vi "LockFP.vi"(8 "error in (no error)":errorcluster, 11 "TektronixDPO_PhysicalDevice in":refnum<class "TektronixDPO_PhysicalDevice.lvclass">) -> (0 "error out":errorcluster, 3 "TektronixDPO_PhysicalDevice out":refnum<class "TektronixDPO_PhysicalDevice.lvclass">)   [LabVIEW 2013, in "TektronixDPO_PhysicalDevice.lvclass"]
uses:
  TektronixDPO_PhysicalDevice.lvclass
  TektronixDPO_PhysicalDevice.lvclass/TektronixDPO_PhysicalDevice.ctl
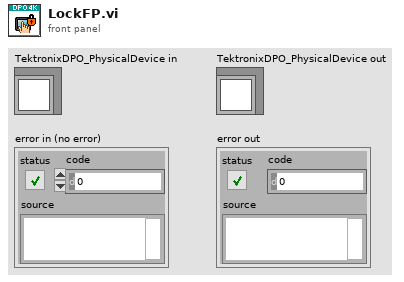
[diagram p1: front panel]
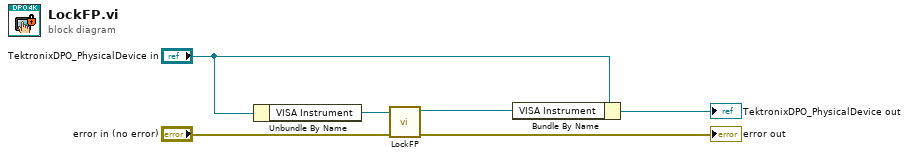
[diagram p0: block diagram]
diagram:
  n1 = Unbundle By Name("TektronixDPO_PhysicalDevice in") -> ("VISA Instrument"=w1:refnum<visa-resource-name>)
  n2 = call "LockFP.vi"("error in (no error)"="error in (no error)", "VISA resource name"=w1) -> ("error out"=→"error out":errorcluster, "VISA resource name out"=w4:refnum<visa-resource-name>)  [unwired: 8 in]
  n3 = Bundle By Name(cluster="TektronixDPO_PhysicalDevice in", "VISA Instrument"=w4) -> (→"TektronixDPO_PhysicalDevice out":refnum<class "TektronixDPO_PhysicalDevice.lvclass">)
